vi "IMAQ LL-Ring.vi"(8 "ErrIn":errorcluster, 11 "IF Name":string="img0") -> (0 "ErrOut":errorcluster, 3 "ImgOut":T1)   [LabVIEW 2013]
doc: "Use this template to build a VI to use as a subVI."
uses:
  <vilib>/vision/Image Controls.llb/IMAQ Image.ctl
panel:
  out "Last Valid Buffer":i32
  in  "Number of buffers":i32=10
  in  "stop":bool
  out "Frame Rate":dbl
  # "Input Parameters"
  # "Output Parameters"
  # "VI Description:\nThis VI is created to snap a image from imaging device."
  # ":: MVI Framework V1.0 ::\nAuthor:Gaoke Yang\nEmail: gaoke.yang@yahoo.com\nWeb: www.mvicontrol.com\nCopyright (C) 2013, MVI Technologies All Rights Reserved"
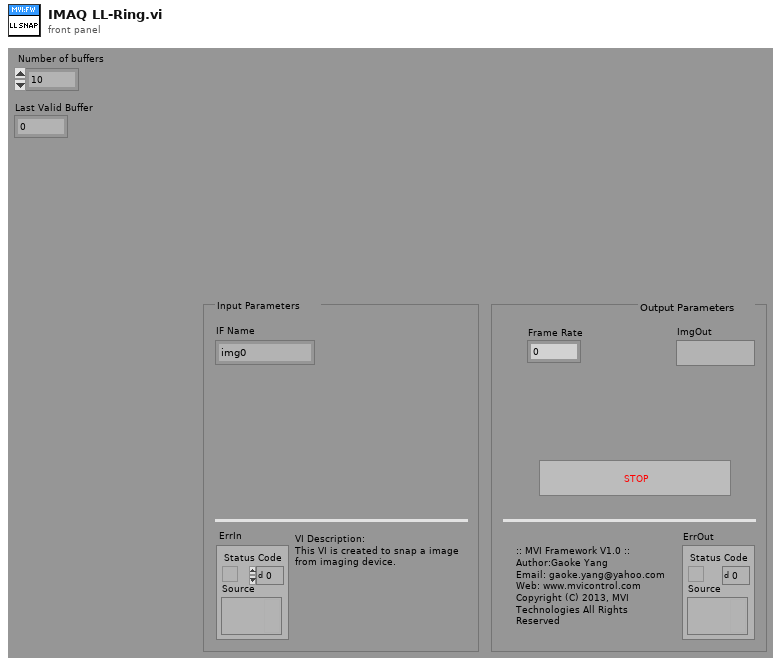
[diagram p1: front panel]
types:
  T1 = typedef "IMAQ Image.ctl" = refnum<image>
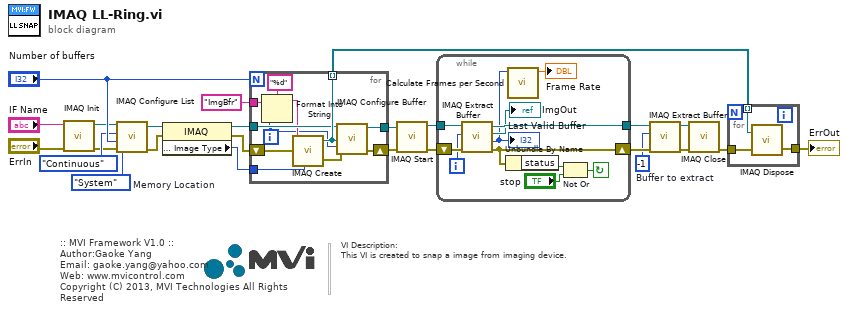
[diagram p0: block diagram]
diagram:
  w7 = -1  # Buffer to extract
  w18 = enum16{"System", "Onboard"}."System"  # Memory Location
  # "VI Description:\nThis VI is created to snap a image from imaging device."
  # ":: MVI Framework V1.0 ::\nAuthor:Gaoke Yang\nEmail: gaoke.yang@yahoo.com\nWeb: www.mvicontrol.com\nCopyright (C) 2013, MVI Technologies All Rights Reserved"
  n1 = call <vilib>:"IMAQ Init.vi"("error in (no error)"="ErrIn", "Interface Name"="IF Name") -> ("error out"=w19:errorcluster, "IMAQ Session Out"=w21:refnum<k11>)  [unwired: 8 out]
  n2 = call <vilib>:"IMAQ Configure List.vi"("Memory Location"=w18, "error in (no error)"=w19, "Number of buffers"="Number of buffers", "Continuous?"=enum16{"One-Shot", "Continuous"}."Continuous" ("Continuous ?"), "IMAQ Session In"=w21) -> ("error out"=w16:errorcluster, "IMAQ Session Out"=w17:refnum<k11>)  [unwired: 1 in, 4 out]
  n3 = property class="IMAQ"(reference=w17, error in=w16) -> (reference out=w4:refnum<k11>, error out=w5:errorcluster, "Image Parameters : Image Type"=w3:u32)
  n4 = for {
    N: "Number of buffers" -> [_]
    tunnel: [w36] -> w14
    tunnel: w3 -> [w34]
    tunnel: w4 -> [w30]
    tunnel: [w31] -> w1 mode=indexing
    shift-right: [w35] -> w15
    shift-left: w5 -> [w33]
    tunnel: "ImgBfr" ("ImgBfr") -> [w26]
    i -> [w28]
    n5 = Format Into String(format string="%d", initial string=w26, w28) -> (resulting string=w29:string)  [unwired: 1 in, 1 out]
    n6 = call "IMAQ Create"("Image Name"=w29, "Image Type"=w34, "error in (no error)"=w33) -> ("New Image"=w31:T1, "error out"=w32:errorcluster)  [unwired: 1 in, 1 out]
    n7 = call <vilib>:"IMAQ Configure Buffer.vi"("error in (no error)"=w32, "Buffer Number"=w28, "Image In"=w31, "IMAQ Session In"=w30) -> ("error out"=w35:errorcluster, "IMAQ Session Out"=w36:refnum<k11>)  [unwired: 2 in, 4 out]
  }
  n8 = call <vilib>:"IMAQ Start.vi"("error in (no error)"=w15, "IMAQ Session In"=w14) -> ("error out"=w10:errorcluster, "IMAQ Session Out"=w11:refnum<k11>)  [unwired: 8 out]
  n9 = while {
    shift-left: w10 -> [w47]
    shift-right: [w39] -> w9
    tunnel: [w45] -> w8
    tunnel: w11 -> [w46]
    i -> [w44]
    stop <- w40 continue-if-true
    n10 = call <vilib>:"IMAQ Extract Buffer.vi"("error in (no error)"=w47, "Buffer to extract"=w44, "IMAQ Session In"=w46) -> ("error out"=w39:errorcluster, "Buffer Number"=w38:i32, "Image Out"=→"ImgOut":T1, "IMAQ Session Out"=w45:refnum<k11>)  [unwired: 5 out]
    "Last Valid Buffer" <- w38
    n11 = Unbundle By Name(w39) -> ("status"=w42:bool)
    n12 = call <vilib>:"Calculate Frames per Second.vi"("Buffer Number"=w38) -> ("Acquired Frames/s"=→"Frame Rate":dbl)  [unwired: 8 in, 2 out]
    n13 = Not Or(1:"stop", 2:w42) -> (0:w40:bool)
  }
  n14 = call <vilib>:"IMAQ Extract Buffer.vi"("error in (no error)"=w9, "Buffer to extract"=w7, "IMAQ Session In"=w8) -> ("error out"=w12:errorcluster, "IMAQ Session Out"=w13:refnum<k11>)  [unwired: 7 out]
  n15 = call <vilib>:"IMAQ Close.vi"("error in (no error)"=w12, "IMAQ Session In"=w13) -> ("error out"=w6:errorcluster)  [unwired: 9 out]
  n16 = for {
    tunnel: w1 -> [w50] mode=indexing
    tunnel: [w48] -> w23
    tunnel: w6 -> [w49]
    n17 = call "IMAQ Dispose"("Image"=w50, "error in (no error)"=w49) -> ("error out"=w48:errorcluster)  [unwired: 1 in, 3 out]
  }
  "ErrOut" <- w23
